vi "Reset Variables.vi"   [LabVIEW 2015]
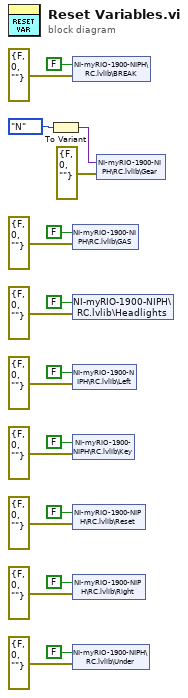
[diagram p0: block diagram]
diagram:
  n1 = To Variant(anything=enum16{"3rd", "2nd", "1st", "N", "R"}."N" ("Enum")) -> (Variant=w1:variant)
  n2 = shared-variable "NI-myRIO-1900-NIPH\\RC.lvlib\\BREAK"(FALSE ("BREAK"), error in=errorcluster {"status"=FALSE, "code"=0, "source"=""} ("error in (no error)")) -> ()  [unwired: 1 out]
  n3 = shared-variable "NI-myRIO-1900-NIPH\\RC.lvlib\\GAS"(FALSE ("GAS"), error in=errorcluster {"status"=FALSE, "code"=0, "source"=""} ("error in (no error)")) -> ()  [unwired: 1 out]
  n4 = shared-variable "NI-myRIO-1900-NIPH\\RC.lvlib\\Headlights"(FALSE ("Headlights"), error in=errorcluster {"status"=FALSE, "code"=0, "source"=""} ("error in (no error)")) -> ()  [unwired: 1 out]
  n5 = shared-variable "NI-myRIO-1900-NIPH\\RC.lvlib\\Left"(FALSE ("Left"), error in=errorcluster {"status"=FALSE, "code"=0, "source"=""} ("error in (no error)")) -> ()  [unwired: 1 out]
  n6 = shared-variable "NI-myRIO-1900-NIPH\\RC.lvlib\\Key"(FALSE ("Key"), error in=errorcluster {"status"=FALSE, "code"=0, "source"=""} ("error in (no error)")) -> ()  [unwired: 1 out]
  n7 = shared-variable "NI-myRIO-1900-NIPH\\RC.lvlib\\Reset"(FALSE ("Reset"), error in=errorcluster {"status"=FALSE, "code"=0, "source"=""} ("error in (no error)")) -> ()  [unwired: 1 out]
  n8 = shared-variable "NI-myRIO-1900-NIPH\\RC.lvlib\\Right"(FALSE ("Right"), error in=errorcluster {"status"=FALSE, "code"=0, "source"=""} ("error in (no error)")) -> ()  [unwired: 1 out]
  n9 = shared-variable "NI-myRIO-1900-NIPH\\RC.lvlib\\Under"(FALSE ("Under"), error in=errorcluster {"status"=FALSE, "code"=0, "source"=""} ("error in (no error)")) -> ()  [unwired: 1 out]
  n10 = shared-variable "NI-myRIO-1900-NIPH\\RC.lvlib\\Gear"(w1, error in=errorcluster {"status"=FALSE, "code"=0, "source"=""} ("error in (no error)")) -> ()  [unwired: 1 out]
